vi "Quiz4.vi"() -> ()   [LabVIEW 2020]
uses:
  <vilib>/Platform/TimedLoop/XDataNode/timing_clust.ctl
  <vilib>/Platform/TimedLoop/XDataNode/nitl_modes.ctl
  <vilib>/Platform/TimedLoop/XDataNode/wakeup.ctl
  Control 1.ctl
  <vilib>/Utility/file.llb/Read Delimited Spreadsheet (string).vi
  <vilib>/platform/TimedLoop/XDataNode/XDataNode.xnode
  <vilib>/Platform/TimedLoop/XDataNode/XDNodeRunTimeDep.lvlib
panel:
  in  "OK Button 4":bool
  in  "OK Button 3":bool
  in  "Tab Control 2":enum32{"Login", "Registro", "Inicio"}(tab)
  in  "OK Button 2":bool
  in  "Clave 2":string
  in  "Usuario 2":string
  in  "Borrar usuario 2":string
  in  "Borrar 2":bool
  in  "Volver 2":bool
  in  "Agregar 2":bool
  in  "Clave Nueva 2":string
  in  "Nuevo Usuario 2":string
  out "concatenated string 2":string
  out "String 2":string="Usuario incorrecto"
  out "Usuarios Eliminados 2":string[](array[string])
  in  "Cerrar sesión 2":bool
  out "Usuarios 2":string[](array[string])
  out "Contraseñas 2":string[](array[string])
  out "Contraseñas":string[](array[string])
  out "Usuarios":string[](array[string])
  in  "Tab Control":enum32{"Login", "Registro", "Inicio"}(tab)
  in  "OK Button":bool
  in  "Clave":string
  in  "Usuario":string
  in  "Borrar usuario":string
  in  "Borrar":bool
  in  "Volver":bool
  in  "Agregar":bool
  in  "Clave Nueva":string
  in  "Nuevo Usuario":string
  out "concatenated string":string
  out "String":string="Usuario incorrecto"
  out "Usuarios Eliminados":string[](array[string])
  in  "Cerrar sesión":bool
  # "Usuario"
  # "Clave"
  # "Nuevo Usuario"
  # "Borrar usuario"
  # "Clave Nueva"
  # "Usuarios Eliminados"
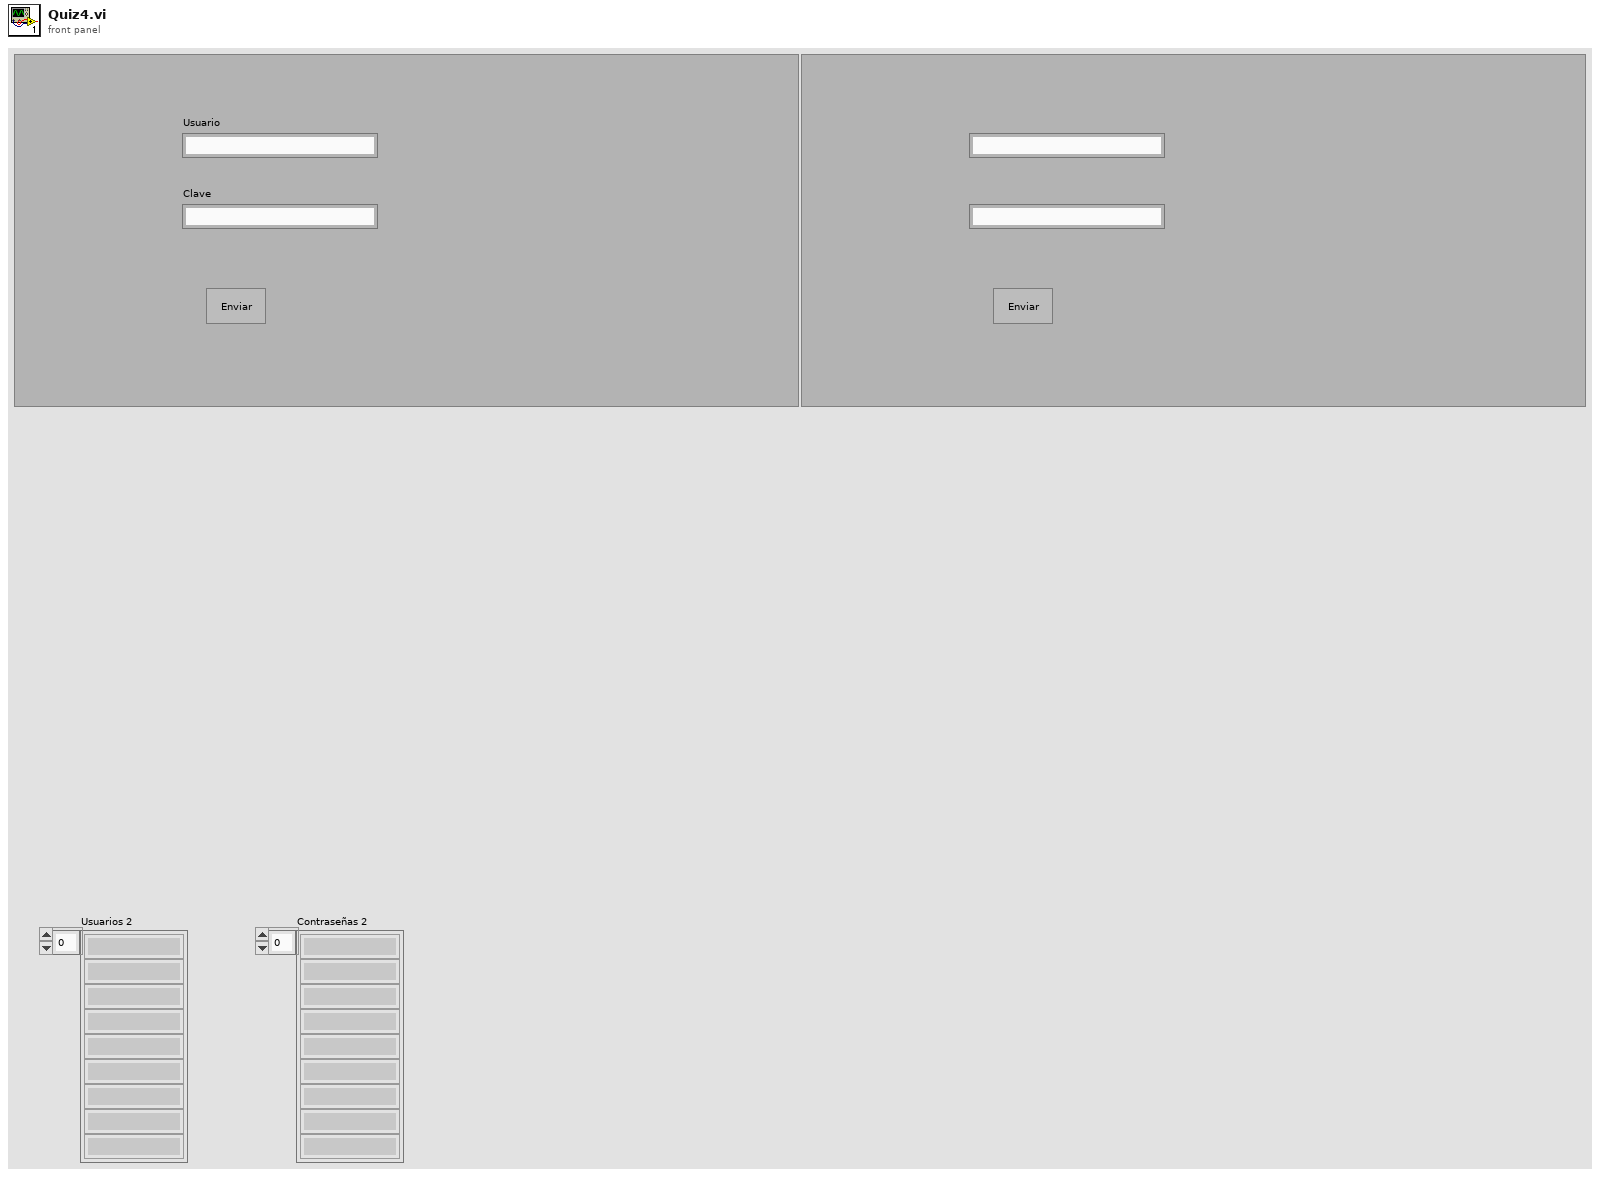
[diagram p1: front panel]
types:
  T1 = typedef "Control 1.ctl" = enum16{"Login", "Registro", "Inicio"}
  T2 = enum16{"open", "replace", "create", "open or create", "replace or create", "replace or create with confirmation"}
  T3 = typedef "XDNodeRunTimeDep.lvlib/timing_clust.ctl" = cluster{"Expected End [f-1]":u64, "Actual End [f-1]":u64, "Finished Late? [f-1]":bool, "Expected End [i-1]":u64, "Actual End [i-1]":u64, "Finished Late? [i-1]":bool, "Expected Start [i]":u64, "Actual Start [i]":u64, "Expected Start [f]":u64, "Actual Start [f]":u64, "Source Name":string, "Structure Name":string, "Period":i64, "Deadline":i64, "Offset":i64, "Start":i64, "Priority":i32, "Timeout":i32, "Mode":T4, "Wakeup Reason":T5, "Error":errorcluster, "Source Type":string, "Secondary Source Type":string, "Global End Time":u64, "Global Start Time":u64, "Frame Duration":u64, "Iteration Duration":u64, "Assigned CPU":i32, "I/O Scan Engine Mode":u32}
  T4 = typedef "XDNodeRunTimeDep.lvlib/nitl_modes.ctl" = enum32{"No Change", "Process missed periods, maintain original phase", "Discard missed periods, maintain original phase", "Process missed periods, ignore original phase", "Discard missed periods, ignore original phase"}
  T5 = typedef "XDNodeRunTimeDep.lvlib/wakeup.ctl" = enum32{"Normal", "Aborted", "Asynchronous wakeup", "Timing source error", "Timed loop error", "Timeout"}
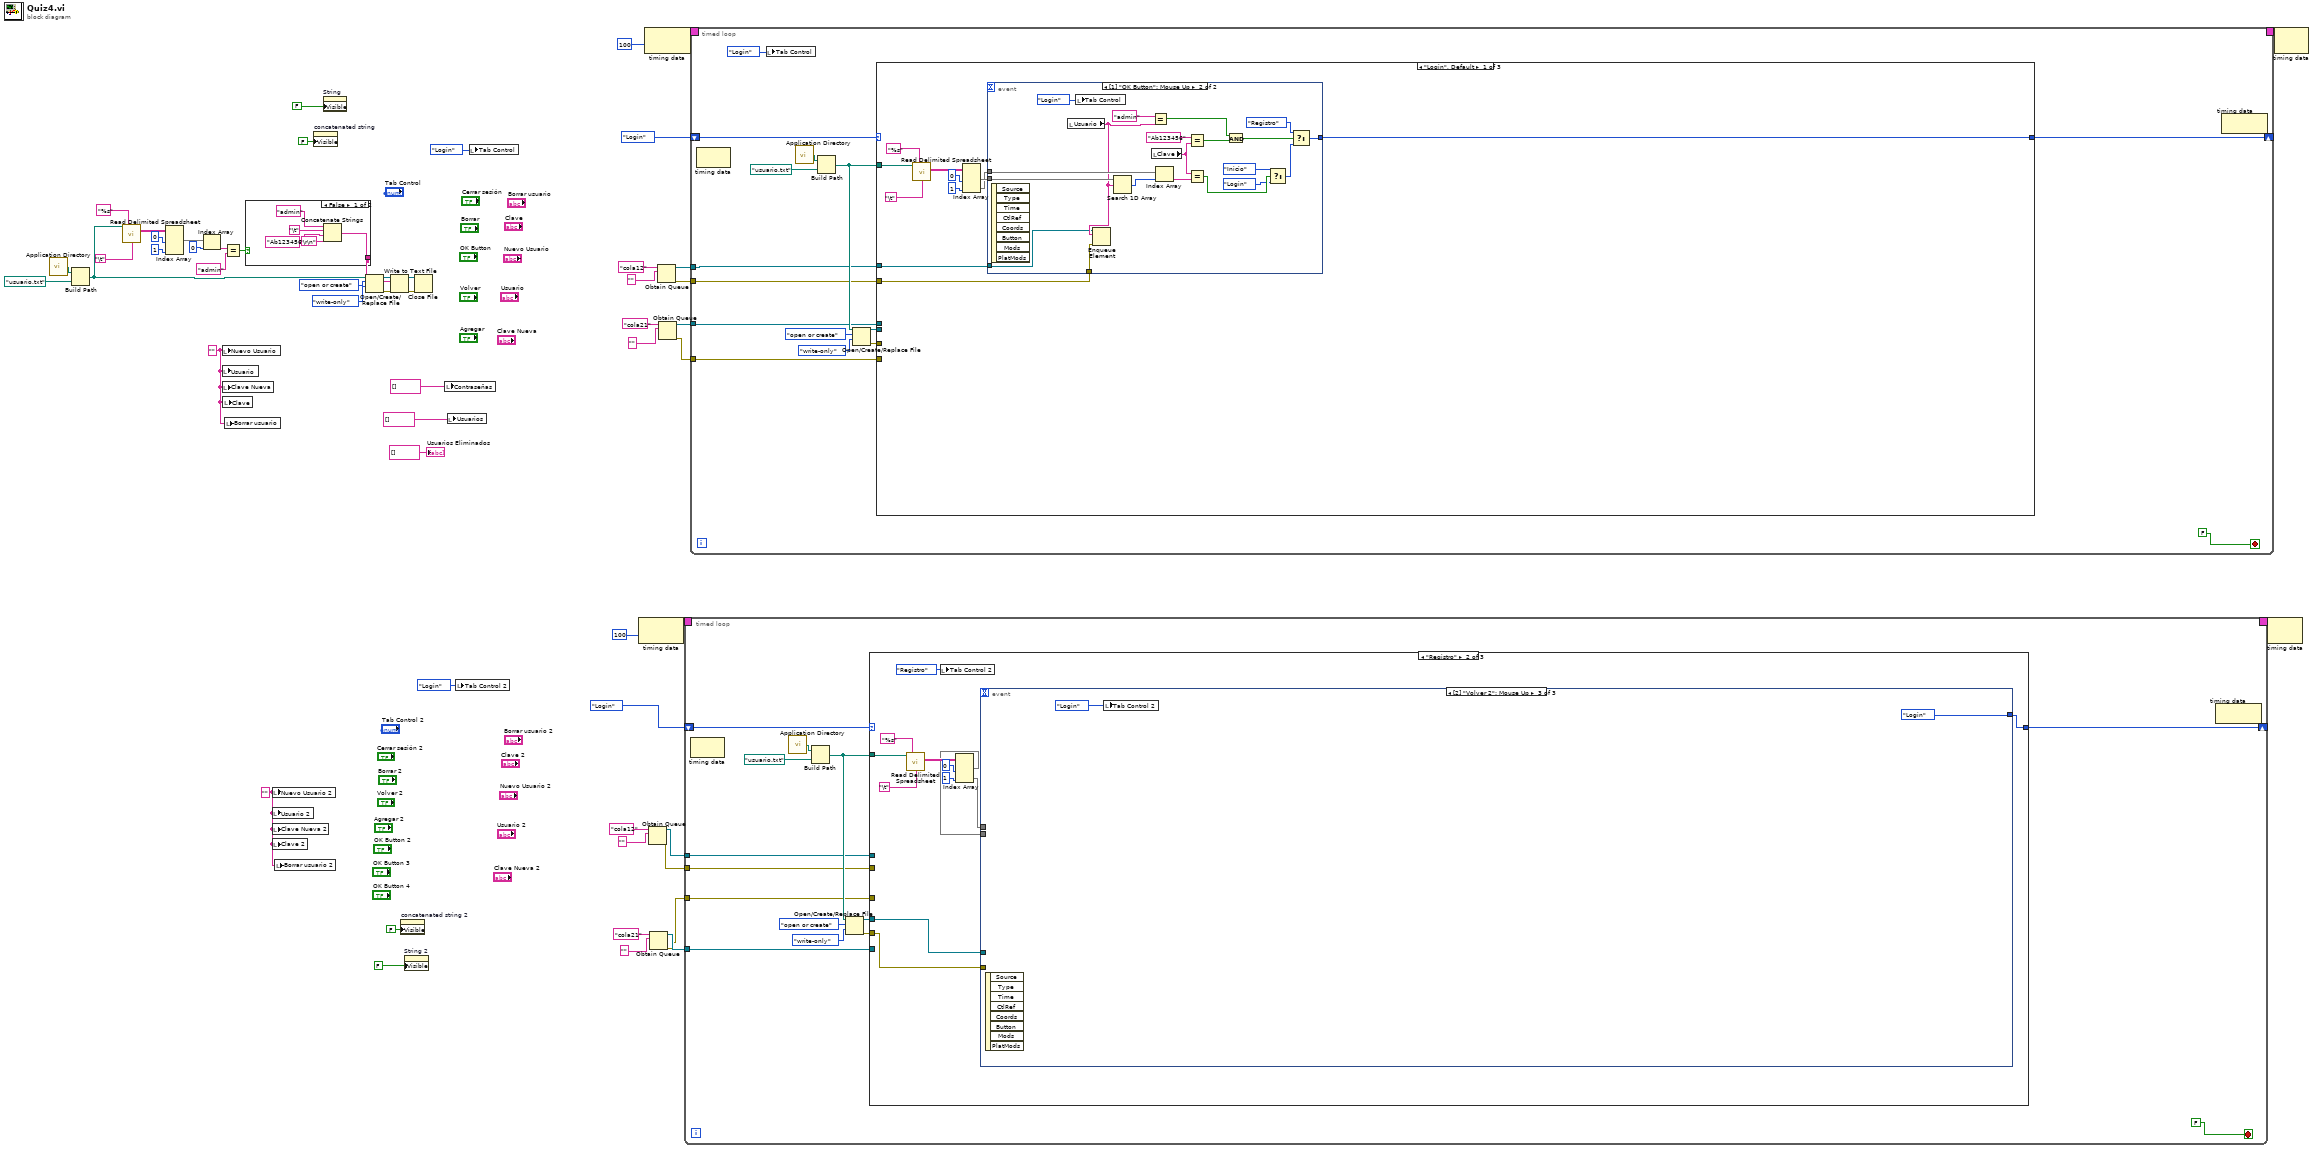
[diagram p0: block diagram]
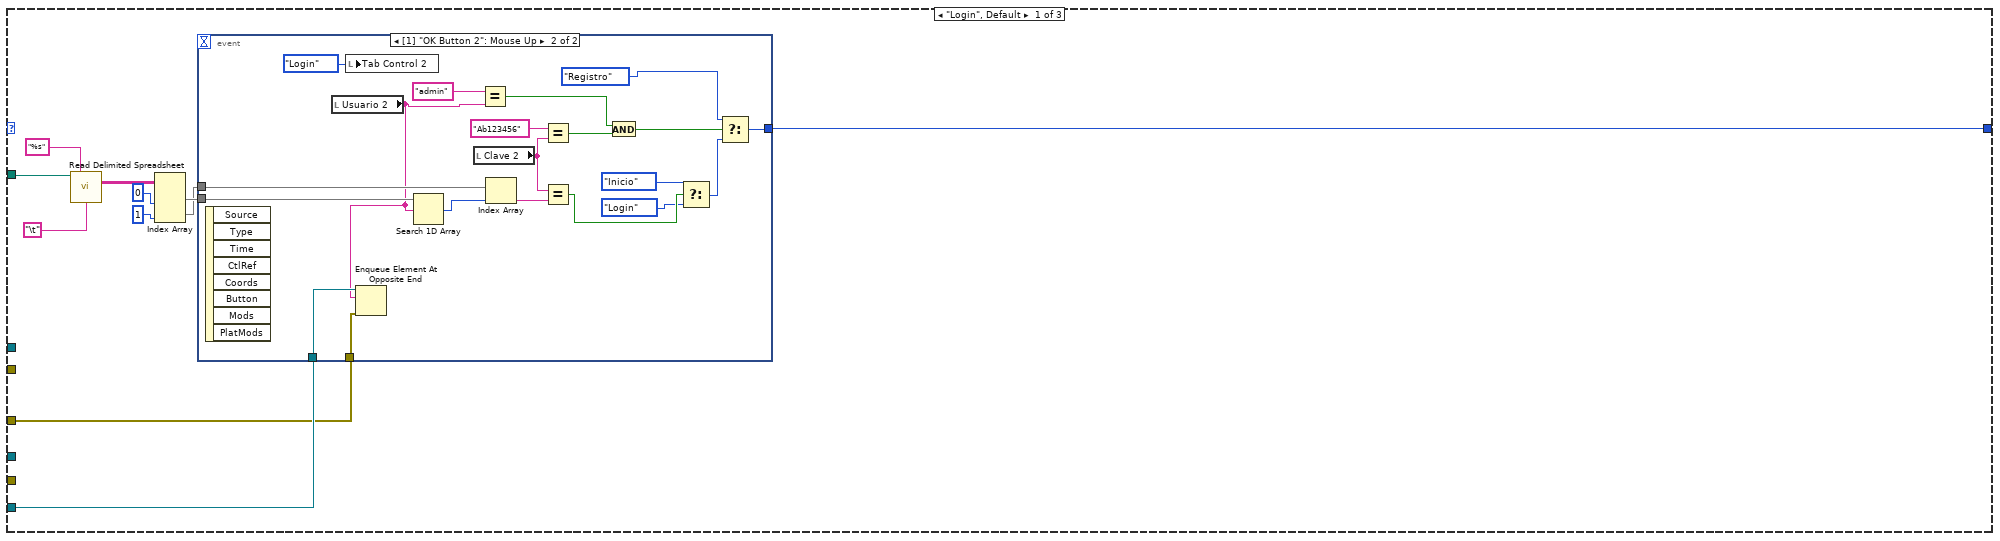
[diagram p2: hidden frame]
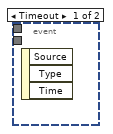
[diagram p3: hidden frame]
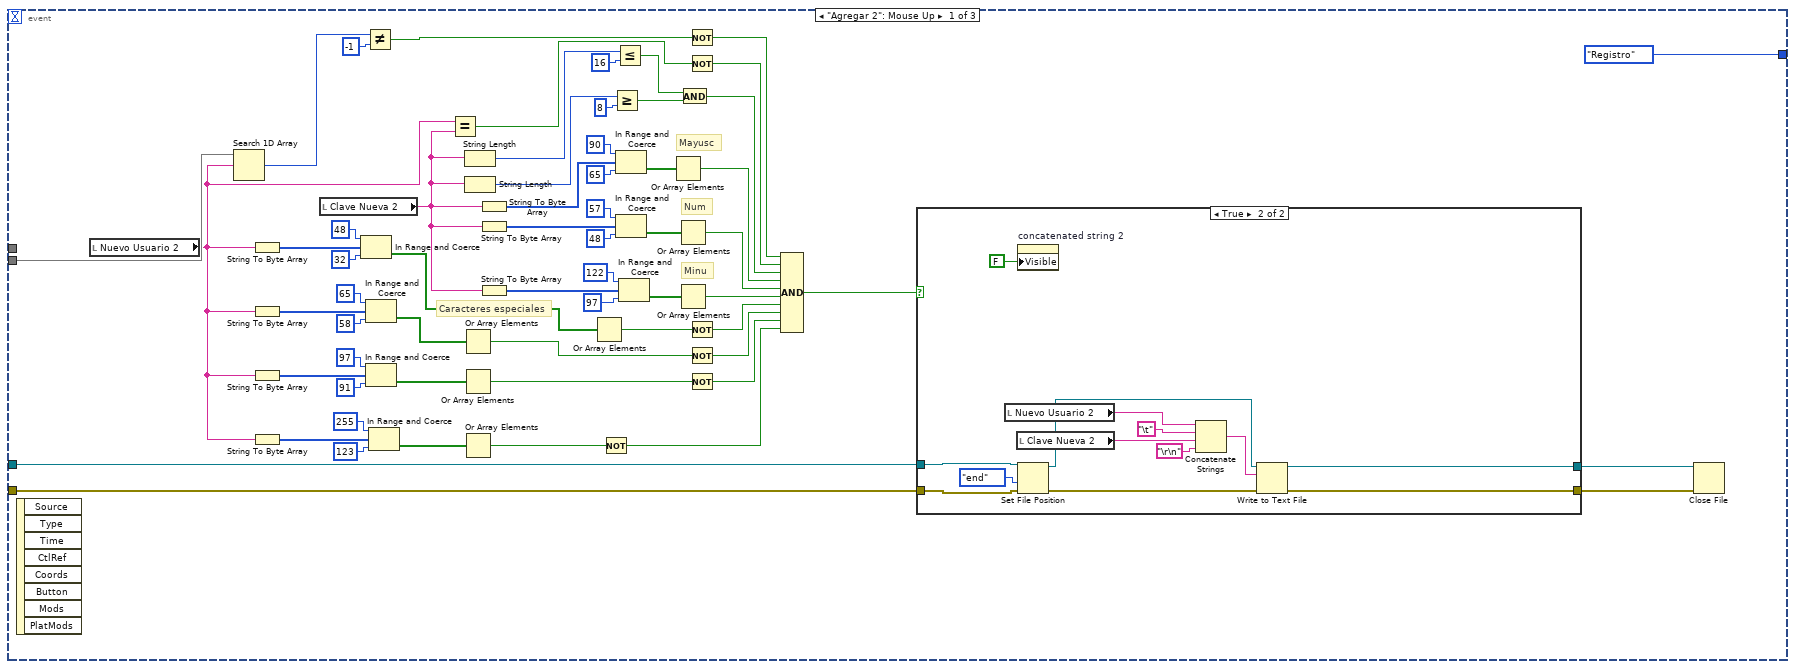
[diagram p4: hidden frame]
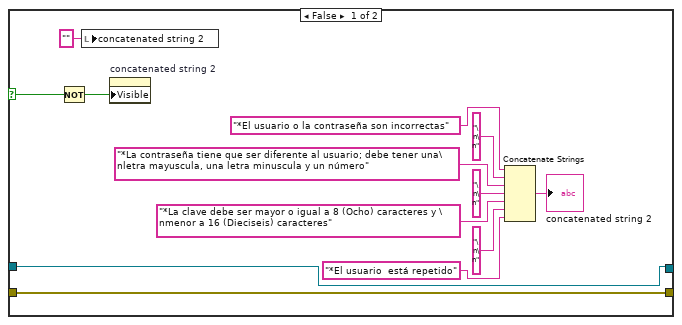
[diagram p5: hidden frame]
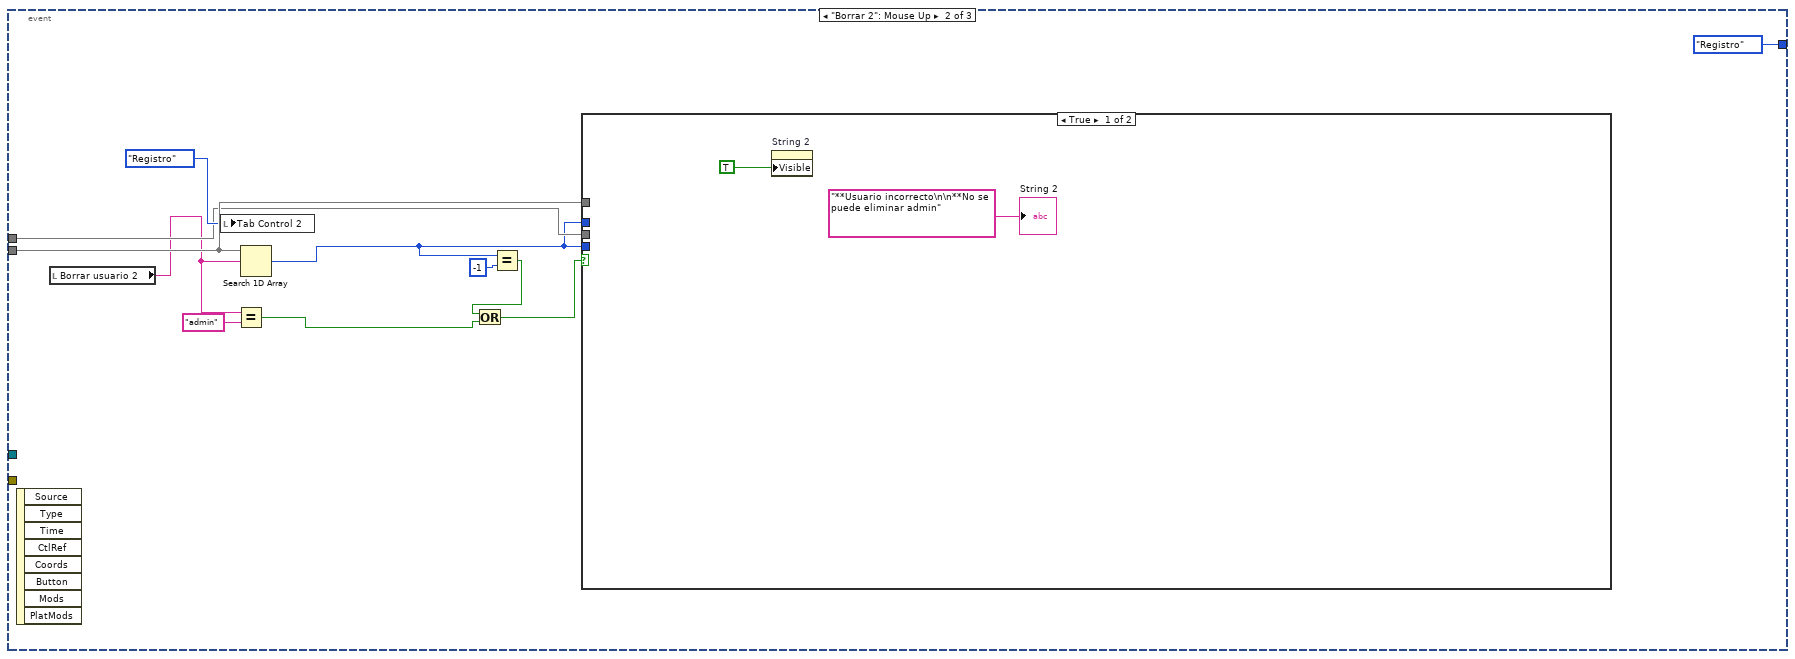
[diagram p6: hidden frame]
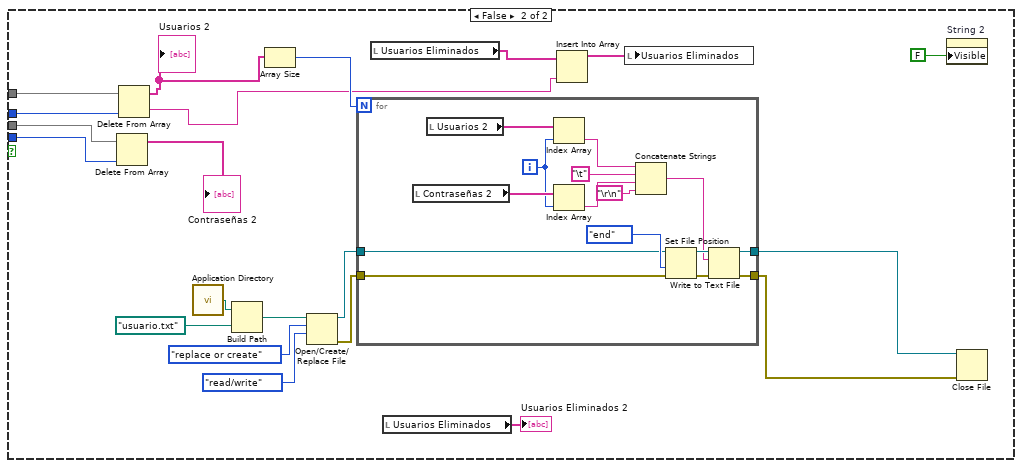
[diagram p7: hidden frame]
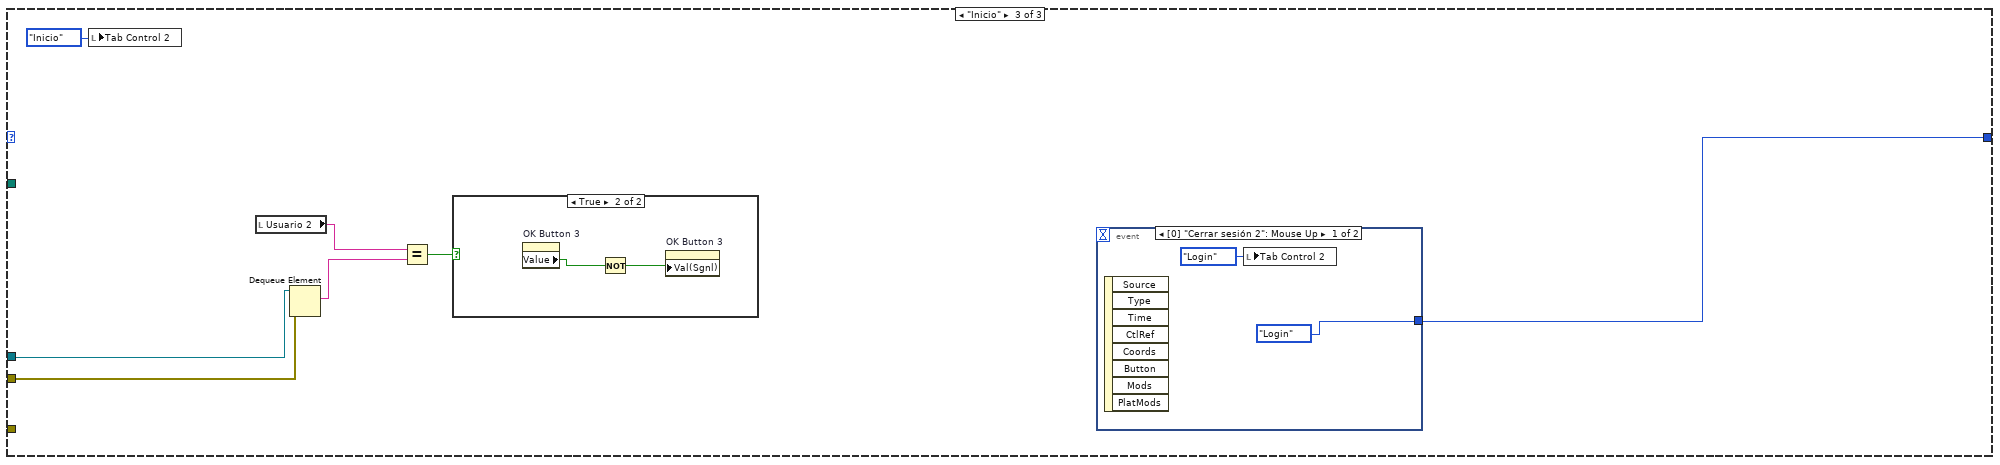
[diagram p8: hidden frame]
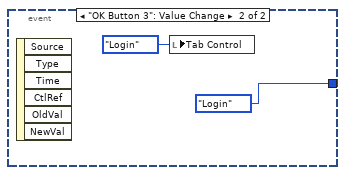
[diagram p10: hidden frame]
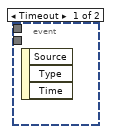
[diagram p12: hidden frame]
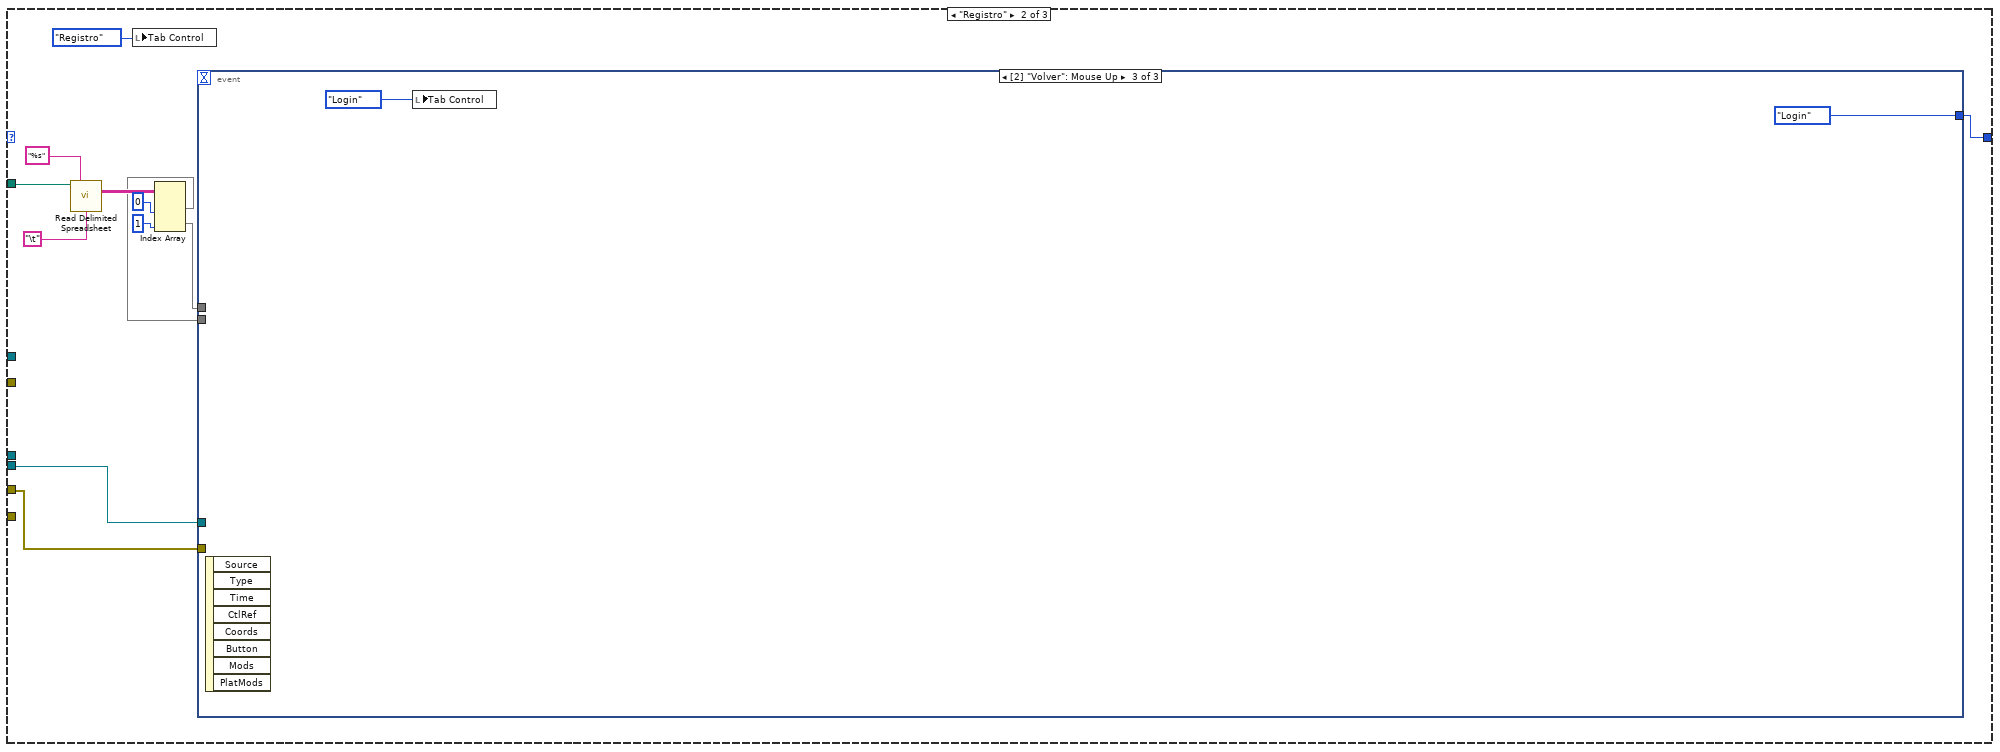
[diagram p13: hidden frame]
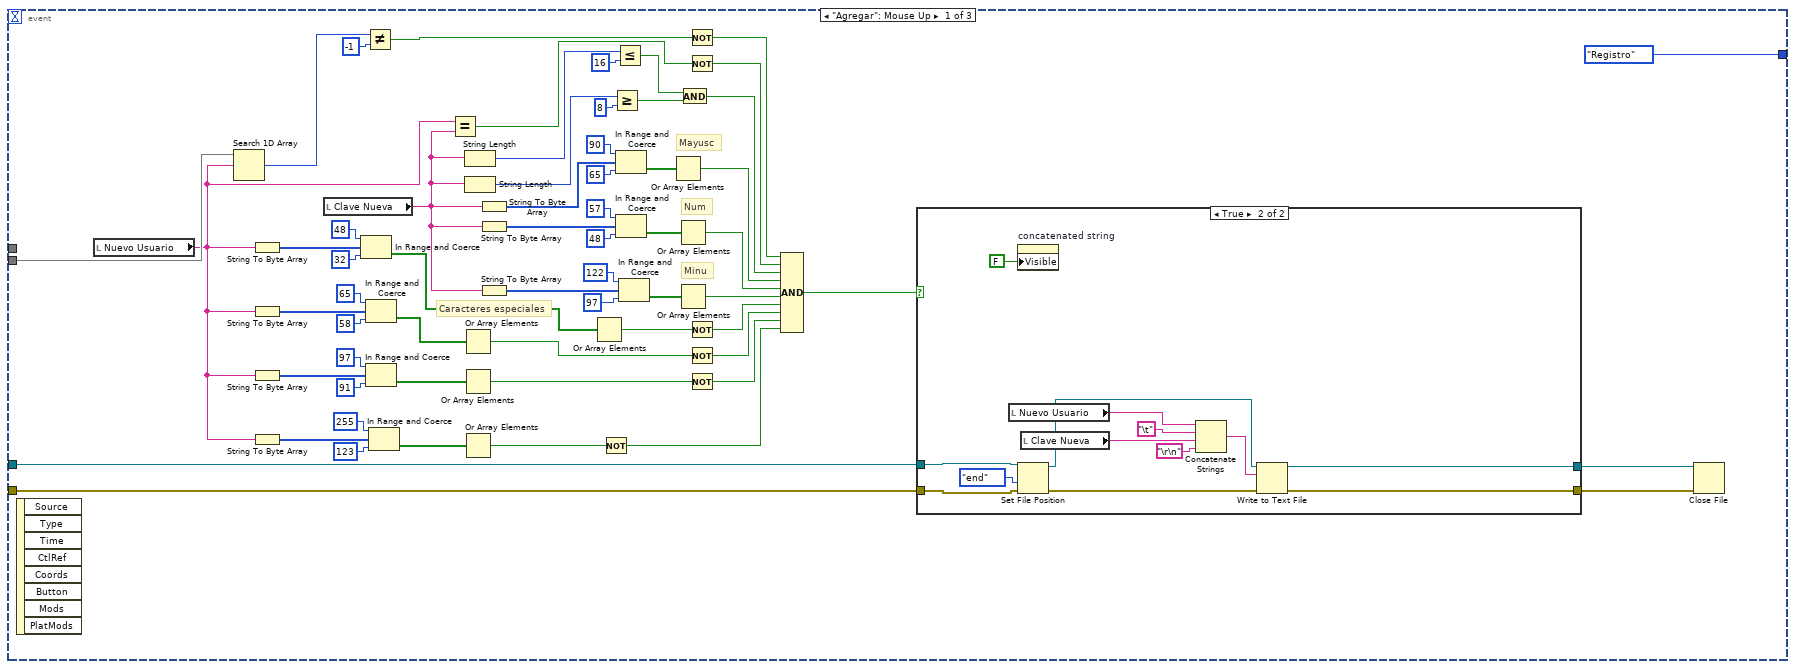
[diagram p14: hidden frame]
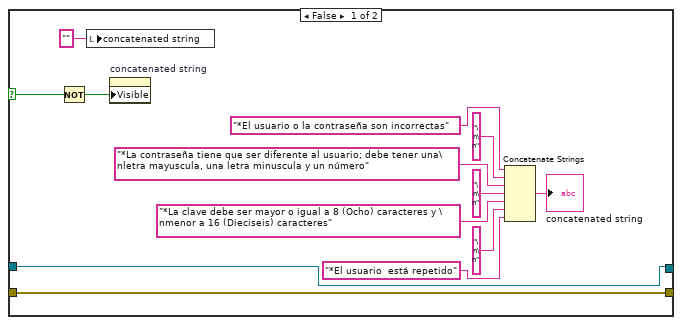
[diagram p15: hidden frame]
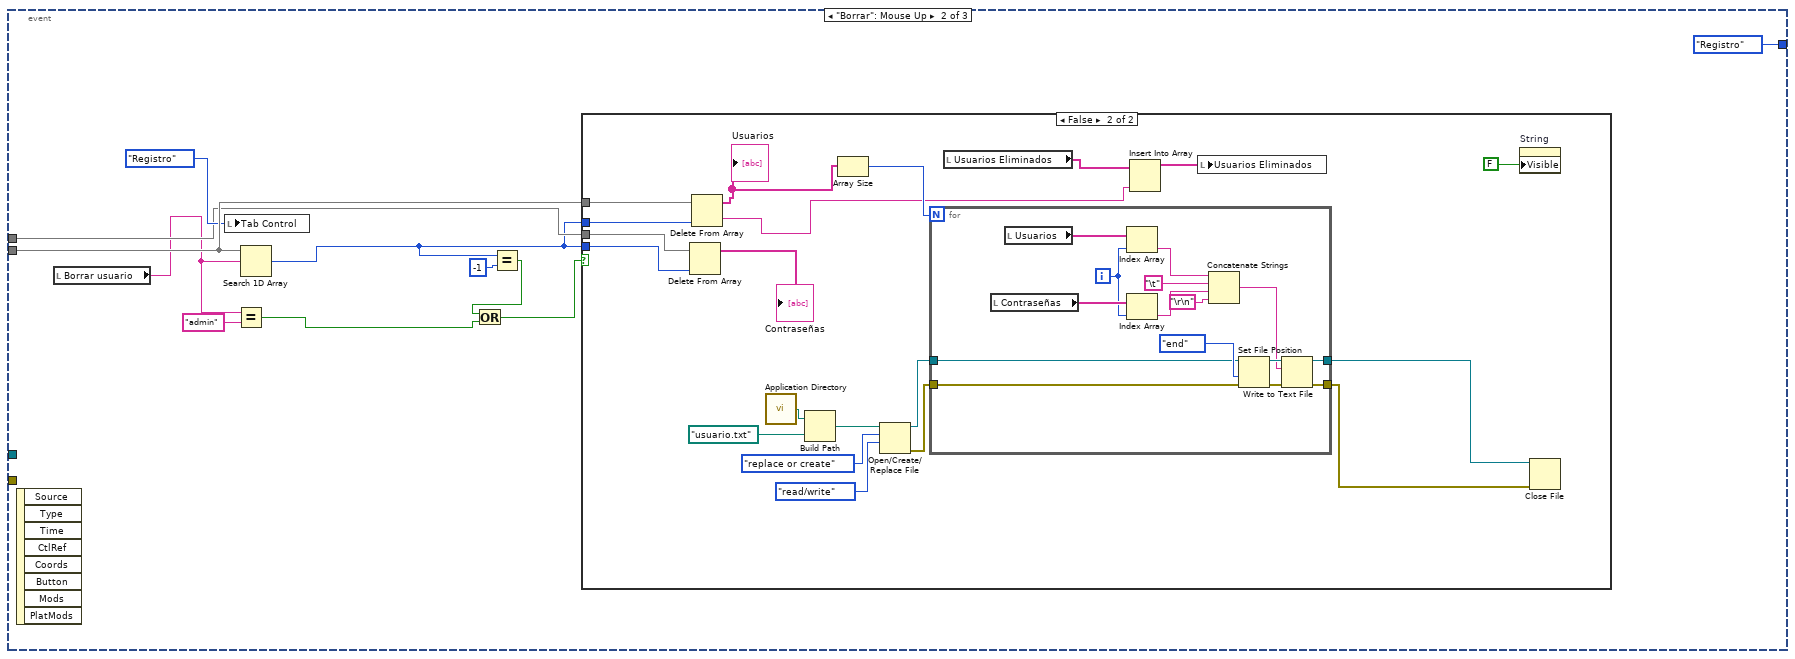
[diagram p16: hidden frame]
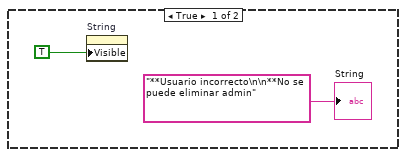
[diagram p17: hidden frame]
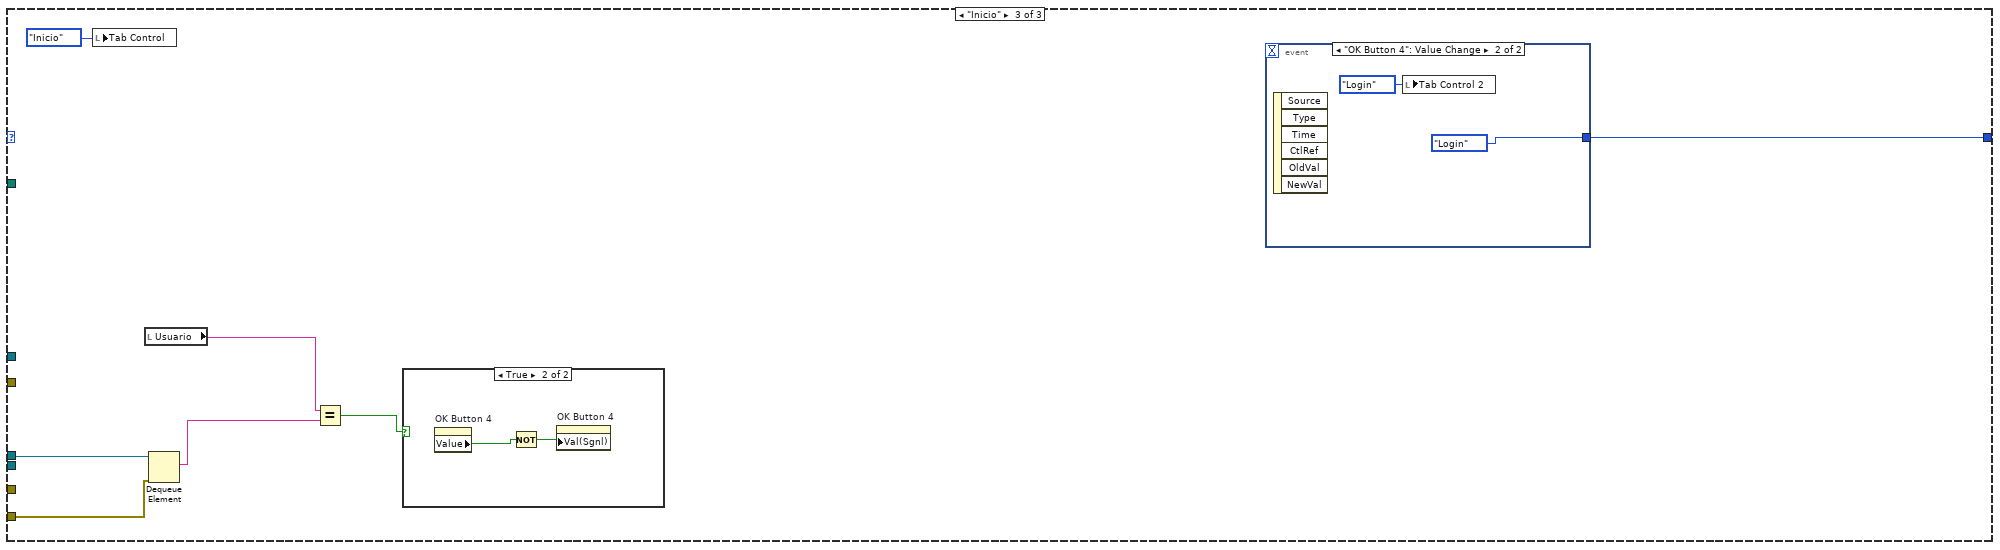
[diagram p18: hidden frame]
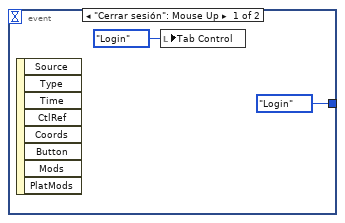
[diagram p20: hidden frame]
diagram:
  w20 = "" ("Nuevo Usuario")
  w25 = "" ("Nuevo Usuario")
  n1 = call <vilib>:"Application Directory.vi"() -> ("Application Directory"=w48:path)
  n2 = Build Path(base path=w48, name or relative path=path "usuario.txt" ("file path (use dialog)")) -> (appended path=w40:path)
  n3 = call-poly <vilib>:"Read Delimited Spreadsheet.vi"("file path (dialog if empty)"=w40, "format (%s)"="%s", "delimiter (\\t)"="\t") -> ("all rows"=w45:string[][])  [unwired: 7 in, 5 out]
  n4 = Index Array(array=w45, index (col) #1=0 ("disabled index (col)"), index (col) #2=1 ("index (col)")) -> (element #1=w39:string[])  [unwired: 2 in, 1 out]
  n5 = Index Array(array=w39, index=0) -> (element=w37:string)
  n6 = local write "Nuevo Usuario"(w25) -> ()
  n7 = local write "Usuario"(w25) -> ()
  n8 = local write "Clave Nueva"(w25) -> ()
  n9 = local write "Clave"(w25) -> ()
  n10 = Equal?(x=w37, y="admin") -> (x = y?=w35:bool)
  n11 = local write "Borrar usuario"(w25) -> ()
  n12 = case shown="False" w35 {
    tunnel: [w56 _] -> w30
    frame False {
      n13 = Concatenate Strings("admin" ("string"), "\t", "Ab123456" ("string"), "\r\n") -> (w56:string)
    }
    frame True {
    }
  }
  n14 = local write "Nuevo Usuario 2"(w20) -> ()
  n15 = local write "Usuario 2"(w20) -> ()
  n16 = local write "Clave Nueva 2"(w20) -> ()
  n17 = local write "Clave 2"(w20) -> ()
  n18 = local write "Borrar usuario 2"(w20) -> ()
  n19 = property on="concatenated string" class="Str"("Visible"=FALSE) -> ()  [unwired: 2 in, 2 out]
  n20 = property on="String" class="Str"("Visible"=FALSE) -> ()  [unwired: 2 in, 2 out]
  n21 = Open/Create/Replace File(file path (use dialog)=w40, operation (0:open)=T2."open or create", access (0:read/write)=enum16{"read/write", "read-only", "write-only"}."write-only") -> (refnum out=w34:refnum<file>, error out=w33:errorcluster)  [unwired: 3 in, 1 out]
  n22 = Write to Text File(file (use dialog)=w34, text=w30, error in=w33) -> (refnum out=w32:refnum<file>, error out=w31:errorcluster)  [unwired: 1 in, 1 out]
  n23 = property on="concatenated string 2" class="Str"("Visible"=FALSE) -> ()  [unwired: 2 in, 2 out]
  n24 = property on="String 2" class="Str"("Visible"=FALSE) -> ()  [unwired: 2 in, 2 out]
  n25 = Close File(refnum=w32, error in=w31) -> ()  [unwired: 2 out]
  n26 = local write "Contraseñas"(string[] [] ("array w/ subset deleted 2")) -> ()
  n27 = local write "Usuarios"(string[] [] ("array w/ subset deleted 2")) -> ()
  n28 = local write "Tab Control 2"(enum32{"Login", "Registro", "Inicio"}."Login" ("Tab Control 2")) -> ()
  n29 = local write "Tab Control"(enum32{"Login", "Registro", "Inicio"}."Login" ("Tab Control")) -> ()
  n30 = node-c288(i64 100 ("Period")) -> (w24:T3)
  n31 = node-c288(i64 100 ("Period")) -> (w55:T3)
  n32 = Obtain Queue(name (unnamed)="cola12", element data type="") -> (queue out=w11:refnum<queue>, error out=w10:errorcluster)  [unwired: 3 in, 1 out]
  n33 = Obtain Queue(name (unnamed)="cola21", element data type="") -> (queue out=w8:refnum<queue>, error out=w7:errorcluster)  [unwired: 3 in, 1 out]
  n34 = Obtain Queue(name (unnamed)="cola12", element data type="") -> (queue out=w15:refnum<queue>, error out=w14:errorcluster)  [unwired: 3 in, 1 out]
  n35 = Obtain Queue(name (unnamed)="cola21", element data type="") -> (queue out=w5:refnum<queue>, error out=w4:errorcluster)  [unwired: 3 in, 1 out]
  n36 = timed-loop {
    timing: w24 -> [_]
    timing-out: [_] -> w23
    shift-right: [w73] -> _
    shift-left: Control_1."Login" -> [w61]
    tunnel: w11 -> [w65]
    tunnel: w10 -> [w64]
    tunnel: w8 -> [w63]
    tunnel: w7 -> [w62]
    stop <- FALSE stop-if-true
    n37 = node-c288() -> ()  [unwired: 1 in, 1 out]
    n38 = call <vilib>:"Application Directory.vi"() -> ("Application Directory"=w71:path)
    n39 = Build Path(base path=w71, name or relative path=path "usuario.txt" ("file path (use dialog)")) -> (appended path=w66:path)
    n40 = Open/Create/Replace File(file path (use dialog)=w66, operation (0:open)=T2."open or create", access (0:read/write)=enum16{"read/write", "read-only", "write-only"}."write-only") -> (refnum out=w69:refnum<file>, error out=w68:errorcluster)  [unwired: 3 in, 1 out]
    n41 = case shown="\"Registro\"" w61 {
      tunnel: [w85 w114 w261] -> w73
      tunnel: w69 -> [_ w116 _]
      tunnel: w68 -> [_ w115 _]
      tunnel: w66 -> [w79 w111 _]
      tunnel: w65 -> [_ _ w260]
      tunnel: w64 -> [_ _ w259]
      tunnel: w63 -> [w76 _ _]
      tunnel: w62 -> [w75 _ _]
      frame "Login", Default {
        n42 = call-poly <vilib>:"Read Delimited Spreadsheet.vi"("file path (dialog if empty)"=w79, "format (%s)"="%s", "delimiter (\\t)"="\t") -> ("all rows"=w80:string[][])  [unwired: 7 in, 5 out]
        n43 = Index Array(array=w80, index (col) #1=0 ("disabled index (col)"), index (col) #2=1 ("index (col)")) -> (element #1=w78:string[], element #2=w77:string[])  [unwired: 2 in]
        n44 = event shown="[1] \"OK Button 2\": Mouse Up" {
          selector: _ -> [_ _]
          dyn-events: _ -> [_ _]
          timeout: _ -> [_ _]
          tunnel: [_ w100] -> w85
          tunnel: w78 -> [_ w98]
          tunnel: w77 -> [_ w97]
          tunnel: w76 -> [_ w89]
          tunnel: w75 -> [_ w88]
          event Timeout {
            n45 = event-data() -> ()  [unwired: 1 in, 3 out]
          }
          event "OK Button 2": Mouse Up {
            n46 = event-data() -> ()  [unwired: 1 in, 8 out]
            n47 = local read "Usuario 2"() -> (w87:string)
            n48 = local write "Tab Control 2"(enum32{"Login", "Registro", "Inicio"}."Login" ("Tab Control")) -> ()
            n49 = Enqueue Element At Opposite End(queue=w89, element=w87, error in (no error)=w88) -> ()  [unwired: 1 in, 3 out]
            n50 = Search 1D Array(1D array=w98, element=w87) -> (index of element=w96:i32)  [unwired: 1 in]
            n51 = local read "Clave 2"() -> (w95:string)
            n52 = Equal?(x="admin", y=w87) -> (x = y?=w103:bool)
            n53 = Index Array(array=w97, index=w96) -> (element=w94:string)
            n54 = Equal?(x="Ab123456", y=w95) -> (x = y?=w102:bool)
            n55 = Equal?(x=w95, y=w94) -> (x = y?=w93:bool)
            n56 = And(x=w103, y=w102) -> (x .and. y?=w101:bool)
            n57 = Select(t=Control_1."Inicio", s=w93, f=Control_1."Login") -> (s? t:f=w90:T1)
            n58 = Select(t=Control_1."Registro", s=w101, f=w90) -> (s? t:f=w100:T1)
          }
        }
      }
      frame "Registro" {
        n59 = call-poly <vilib>:"Read Delimited Spreadsheet.vi"("file path (dialog if empty)"=w111, "format (%s)"="%s", "delimiter (\\t)"="\t") -> ("all rows"=w108:string[][])  [unwired: 7 in, 5 out]
        n60 = local write "Tab Control 2"(enum32{"Login", "Registro", "Inicio"}."Registro" ("Tab Control")) -> ()
        n61 = Index Array(array=w108, index (col) #1=0 ("disabled index (col)"), index (col) #2=1 ("index (col)")) -> (element #1=w107:string[], element #2=w106:string[])  [unwired: 2 in]
        n62 = event shown="[2] \"Volver 2\": Mouse Up" {
          selector: _ -> [_ _ _]
          dyn-events: _ -> [_ _ _]
          timeout: _ -> [_ _ _]
          tunnel: w116 -> [w151 _ _]
          tunnel: w115 -> [w150 _ _]
          tunnel: [Control_1."Registro" Control_1."Registro" Control_1."Login"] -> w114
          tunnel: w107 -> [w147 w215 _]
          tunnel: w106 -> [_ w212 _]
          event "Agregar 2": Mouse Up {
            # "Caracteres especiales"
            # "Minu"
            # "Num"
            # "Mayusc"
            n63 = event-data() -> ()  [unwired: 1 in, 8 out]
            n64 = local read "Nuevo Usuario 2"() -> (w126:string)
            n65 = Search 1D Array(1D array=w147, element=w126) -> (index of element=w146:i32)  [unwired: 1 in]
            n66 = String To Byte Array(string=w126) -> (unsigned byte array=w142:u8[])
            n67 = String To Byte Array(string=w126) -> (unsigned byte array=w137:u8[])
            n68 = String To Byte Array(string=w126) -> (unsigned byte array=w136:u8[])
            n69 = String To Byte Array(string=w126) -> (unsigned byte array=w127:u8[])
            n70 = local read "Clave Nueva 2"() -> (w148:string)
            n71 = In Range and Coerce(upper limit=u8 48, x=w142, lower limit=u8 32) -> (In Range?=w133:bool[])  [unwired: 1 out]
            n72 = Not Equal?(x=w146, y=-1) -> (x != y?=w144:bool)
            n73 = In Range and Coerce(upper limit=u8 65, x=w137, lower limit=u8 58) -> (In Range?=w132:bool[])  [unwired: 1 out]
            n74 = In Range and Coerce(upper limit=u8 97, x=w136, lower limit=u8 91) -> (In Range?=w131:bool[])  [unwired: 1 out]
            n75 = In Range and Coerce(upper limit=u8 255, x=w127, lower limit=u8 123) -> (In Range?=w130:bool[])  [unwired: 1 out]
            n76 = Equal?(x=w126, y=w148) -> (x = y?=w156:bool)
            n77 = Or Array Elements(Boolean array=w132) -> (logical OR=w124:bool)
            n78 = Or Array Elements(Boolean array=w131) -> (logical OR=w123:bool)
            n79 = Or Array Elements(Boolean array=w130) -> (logical OR=w122:bool)
            n80 = String Length(string=w148) -> (length=w178:i32)
            n81 = String Length(string=w148) -> (length=w176:i32)
            n82 = String To Byte Array(string=w148) -> (unsigned byte array=w164:u8[])
            n83 = String To Byte Array(string=w148) -> (unsigned byte array=w165:u8[])
            n84 = String To Byte Array(string=w148) -> (unsigned byte array=w172:u8[])
            n85 = Or Array Elements(Boolean array=w133) -> (logical OR=w125:bool)
            n86 = Not(x=w122) -> (.not. x?=w118:bool)
            n87 = Greater Or Equal?(x=w176, y=8) -> (x >= y?=w173:bool)
            n88 = Less Or Equal?(x=w178, y=16) -> (x <= y?=w174:bool)
            n89 = In Range and Coerce(upper limit=u8 90, x=w164, lower limit=u8 65) -> (In Range?=w161:bool[])  [unwired: 1 out]
            n90 = In Range and Coerce(upper limit=u8 57, x=w165, lower limit=u8 48) -> (In Range?=w168:bool[])  [unwired: 1 out]
            n91 = In Range and Coerce(upper limit=u8 122, x=w172, lower limit=u8 97) -> (In Range?=w169:bool[])  [unwired: 1 out]
            n92 = Or Array Elements(Boolean array=w161) -> (logical OR=w159:bool)
            n93 = Or Array Elements(Boolean array=w168) -> (logical OR=w158:bool)
            n94 = Or Array Elements(Boolean array=w169) -> (logical OR=w157:bool)
            n95 = And(x=w174, y=w173) -> (x .and. y?=w160:bool)
            n96 = Not(x=w144) -> (.not. x?=w143:bool)
            n97 = Not(x=w156) -> (.not. x?=w155:bool)
            n98 = Not(x=w125) -> (.not. x?=w121:bool)
            n99 = Not(x=w124) -> (.not. x?=w120:bool)
            n100 = Not(x=w123) -> (.not. x?=w119:bool)
            n101 = Compound Arithmetic op=AND(w143, w155, w160, w159, w158, w157, w121, w120, w119, w118) -> (w154:bool)
            n102 = case shown="True" w154 {
              selector: w154 -> [w187 _]
              tunnel: [w182 w196] -> w153
              tunnel: [w181 w195] -> w152
              tunnel: w151 -> [w182 w193]
              tunnel: w150 -> [w181 w192]
              frame False {
                n103 = Not(x=w187) -> (.not. x?=w186:bool)
                n104 = local write "concatenated string 2"("" ("concatenated string")) -> ()
                n105 = property on="concatenated string 2" class="Str"("Visible"=w186) -> ()  [unwired: 2 in, 2 out]
                n106 = Concatenate Strings("*El usuario o la contraseña son incorrectas", "\n\n" ("string"), "*La contraseña tiene que ser diferente al usuario; debe tener una\nletra mayuscula, una letra minuscula y un número", "\n\n" ("string"), "*La clave debe ser mayor o igual a 8 (Ocho) caracteres y \nmenor a 16 (Dieciseis) caracteres", "\n\n" ("string"), "*El usuario  está repetido") -> (→"concatenated string 2":string)
              }
              frame True {
                n107 = local read "Nuevo Usuario 2"() -> (w199:string)
                n108 = local read "Clave Nueva 2"() -> (w200:string)
                n109 = property on="concatenated string 2" class="Str"("Visible"=FALSE) -> ()  [unwired: 2 in, 2 out]
                n110 = Set File Position(refnum=w193, from (0:start)=enum16{"start", "end", "current"}."end", error in=w192) -> (refnum out=w197:refnum<file>, error out=w202:errorcluster)  [unwired: 1 in]
                n111 = Concatenate Strings(w199, "\t", w200, "\r\n") -> (w203:string)
                n112 = Write to Text File(file (use dialog)=w197, text=w203, error in=w202) -> (refnum out=w196:refnum<file>, error out=w195:errorcluster)  [unwired: 1 in, 1 out]
              }
            }
            n113 = Close File(refnum=w153, error in=w152) -> ()  [unwired: 2 out]
          }
          event "Borrar 2": Mouse Up {
            n114 = event-data() -> ()  [unwired: 1 in, 8 out]
            n115 = local read "Borrar usuario 2"() -> (w205:string)
            n116 = local write "Tab Control 2"(enum32{"Login", "Registro", "Inicio"}."Registro" ("Tab Control")) -> ()
            n117 = Equal?(x=w205, y="admin") -> (x = y?=w206:bool)
            n118 = Search 1D Array(1D array=w215, element=w205) -> (index of element=w210:i32)  [unwired: 1 in]
            n119 = Equal?(x=w210, y=-1) -> (x = y?=w208:bool)
            n120 = Or(x=w208, y=w206) -> (x .or. y?=w207:bool)
            n121 = case shown="True" w207 {
              tunnel: w215 -> [_ w238]
              tunnel: w212 -> [_ w237]
              tunnel: w210 -> [_ w236]
              tunnel: w210 -> [_ w235]
              frame True {
                n122 = property on="String 2" class="Str"("Visible"=TRUE) -> ()  [unwired: 2 in, 2 out]
                "String 2" <- "**Usuario incorrecto\n\n**No se puede eliminar admin"
              }
              frame False {
                n123 = Delete From Array(array=w237, index=w236) -> (array with subset deleted=→"Contraseñas 2":string[])  [unwired: 1 in, 1 out]
                n124 = Delete From Array(array=w238, index=w235) -> (deleted portion=w220:string, array with subset deleted=w232:string[])  [unwired: 1 in]
                "Usuarios 2" <- w232
                n125 = call <vilib>:"Application Directory.vi"() -> ("Application Directory"=w225:path)
                n126 = Build Path(base path=w225, name or relative path=path "usuario.txt" ("file path (use dialog)")) -> (appended path=w226:path)
                n127 = Array Size(array=w232) -> (size(s)=w231:i32)
                n128 = Open/Create/Replace File(file path (use dialog)=w226, operation (0:open)=T2."replace or create", access (0:read/write)=enum16{"read/write", "read-only", "write-only"}."read/write") -> (refnum out=w223:refnum<file>, error out=w222:errorcluster)  [unwired: 3 in, 1 out]
                n129 = for {
                  N: w231 -> [_]
                  tunnel: [w242] -> w229
                  tunnel: [w241] -> w230
                  tunnel: w223 -> [w240]
                  tunnel: w222 -> [w239]
                  i -> [w251]
                  n130 = local read "Contraseñas 2"() -> (w252:string[])
                  n131 = local read "Usuarios 2"() -> (w253:string[])
                  n132 = Index Array(array=w253, index=w251) -> (element=w244:string)
                  n133 = Index Array(array=w252, index=w251) -> (element=w243:string)
                  n134 = Concatenate Strings(w244, "\t", w243, "\r\n") -> (w246:string)
                  n135 = Set File Position(refnum=w240, from (0:start)=enum16{"start", "end", "current"}."end", error in=w239) -> (refnum out=w248:refnum<file>, error out=w250:errorcluster)  [unwired: 1 in]
                  n136 = Write to Text File(file (use dialog)=w248, text=w246, error in=w250) -> (refnum out=w241:refnum<file>, error out=w242:errorcluster)  [unwired: 1 in, 1 out]
                }
                n137 = local read "Usuarios Eliminados"() -> (w221:string[])
                n138 = local read "Usuarios Eliminados"() -> (→"Usuarios Eliminados 2":string[])
                n139 = Insert Into Array(array=w221, new element=w220) -> (w219:string[])  [unwired: 1 in]
                n140 = local write "Usuarios Eliminados"(w219) -> ()
                n141 = property on="String 2" class="Str"("Visible"=FALSE) -> ()  [unwired: 2 in, 2 out]
                n142 = Close File(refnum=w230, error in=w229) -> ()  [unwired: 2 out]
              }
            }
          }
          event "Volver 2": Mouse Up {
            n143 = event-data() -> ()  [unwired: 1 in, 8 out]
            n144 = local write "Tab Control 2"(enum32{"Login", "Registro", "Inicio"}."Login" ("Tab Control")) -> ()
          }
        }
      }
      frame "Inicio" {
        n145 = local write "Tab Control 2"(enum32{"Login", "Registro", "Inicio"}."Inicio" ("Tab Control")) -> ()
        n146 = local read "Usuario 2"() -> (w258:string)
        n147 = Dequeue Element(queue=w260, error in (no error)=w259) -> (element=w257:string)  [unwired: 1 in, 3 out]
        n148 = Equal?(x=w258, y=w257) -> (x = y?=w256:bool)
        n149 = case shown="True" w256 {
          frame False {
          }
          frame True {
            n150 = property on="OK Button 3" class="Bool (strict)"() -> ("Value"=w264:bool)  [unwired: 2 in, 2 out]
            n151 = Not(x=w264) -> (.not. x?=w263:bool)
            n152 = property on="OK Button 3" class="Bool (strict)"("Val(Sgnl)"=w263) -> ()  [unwired: 2 in, 2 out]
          }
        }
        n153 = event shown="[0] \"Cerrar sesión 2\": Mouse Up" {
          selector: _ -> [_ _]
          dyn-events: _ -> [_ _]
          timeout: _ -> [_ _]
          tunnel: [Control_1."Login" Control_1."Login"] -> w261
          event "Cerrar sesión 2": Mouse Up {
            n154 = event-data() -> ()  [unwired: 1 in, 8 out]
            n155 = local write "Tab Control 2"(enum32{"Login", "Registro", "Inicio"}."Login" ("Tab Control")) -> ()
          }
          event "OK Button 3": Value Change {
            n156 = event-data() -> ()  [unwired: 1 in, 6 out]
            n157 = local write "Tab Control"(enum32{"Login", "Registro", "Inicio"}."Login" ("Tab Control")) -> ()
          }
        }
      }
    }
    n158 = node-c288() -> ()  [unwired: 1 in, 1 out]
  }
  n159 = timed-loop {
    timing: w55 -> [_]
    timing-out: [_] -> w54
    shift-right: [w283] -> _
    shift-left: Control_1."Login" -> [w284]
    tunnel: w15 -> [w275]
    tunnel: w14 -> [w274]
    tunnel: w5 -> [w273]
    tunnel: w4 -> [w272]
    stop <- FALSE stop-if-true
    n160 = node-c288() -> ()  [unwired: 1 in, 1 out]
    n161 = local write "Tab Control"(enum32{"Login", "Registro", "Inicio"}."Login" ("Tab Control")) -> ()
    n162 = call <vilib>:"Application Directory.vi"() -> ("Application Directory"=w281:path)
    n163 = Build Path(base path=w281, name or relative path=path "usuario.txt" ("file path (use dialog)")) -> (appended path=w276:path)
    n164 = Open/Create/Replace File(file path (use dialog)=w276, operation (0:open)=T2."open or create", access (0:read/write)=enum16{"read/write", "read-only", "write-only"}."write-only") -> (refnum out=w279:refnum<file>, error out=w278:errorcluster)  [unwired: 3 in, 1 out]
    n165 = case shown="\"Login\", Default" w284 {
      tunnel: [w296 w325 w471] -> w283
      tunnel: w279 -> [_ w327 _]
      tunnel: w278 -> [_ w326 _]
      tunnel: w276 -> [w290 w322 _]
      tunnel: w275 -> [w287 _ _]
      tunnel: w274 -> [w286 _ _]
      tunnel: w273 -> [_ _ w470]
      tunnel: w272 -> [_ _ w469]
      frame "Login", Default {
        n166 = call-poly <vilib>:"Read Delimited Spreadsheet.vi"("file path (dialog if empty)"=w290, "format (%s)"="%s", "delimiter (\\t)"="\t") -> ("all rows"=w291:string[][])  [unwired: 7 in, 5 out]
        n167 = Index Array(array=w291, index (col) #1=0 ("disabled index (col)"), index (col) #2=1 ("index (col)")) -> (element #1=w289:string[], element #2=w288:string[])  [unwired: 2 in]
        n168 = event shown="[1] \"OK Button\": Mouse Up" {
          selector: _ -> [_ _]
          dyn-events: _ -> [_ _]
          timeout: _ -> [_ _]
          tunnel: [_ w310] -> w296
          tunnel: w289 -> [_ w308]
          tunnel: w288 -> [_ w307]
          tunnel: w287 -> [_ w298]
          tunnel: w286 -> [_ w297]
          event Timeout {
            n169 = event-data() -> ()  [unwired: 1 in, 3 out]
          }
          event "OK Button": Mouse Up {
            n170 = event-data() -> ()  [unwired: 1 in, 8 out]
            n171 = local read "Usuario"() -> (w299:string)
            n172 = local write "Tab Control"(enum32{"Login", "Registro", "Inicio"}."Login" ("Tab Control")) -> ()
            n173 = Enqueue Element(queue=w298, element=w299, error in (no error)=w297) -> ()  [unwired: 1 in, 3 out]
            n174 = Search 1D Array(1D array=w308, element=w299) -> (index of element=w306:i32)  [unwired: 1 in]
            n175 = local read "Clave"() -> (w305:string)
            n176 = Equal?(x="admin", y=w299) -> (x = y?=w314:bool)
            n177 = Index Array(array=w307, index=w306) -> (element=w304:string)
            n178 = Equal?(x="Ab123456", y=w305) -> (x = y?=w313:bool)
            n179 = Equal?(x=w305, y=w304) -> (x = y?=w303:bool)
            n180 = And(x=w314, y=w313) -> (x .and. y?=w312:bool)
            n181 = Select(t=Control_1."Inicio", s=w303, f=Control_1."Login") -> (s? t:f=w300:T1)
            n182 = Select(t=Control_1."Registro", s=w312, f=w300) -> (s? t:f=w310:T1)
          }
        }
      }
      frame "Registro" {
        n183 = call-poly <vilib>:"Read Delimited Spreadsheet.vi"("file path (dialog if empty)"=w322, "format (%s)"="%s", "delimiter (\\t)"="\t") -> ("all rows"=w319:string[][])  [unwired: 7 in, 5 out]
        n184 = local write "Tab Control"(enum32{"Login", "Registro", "Inicio"}."Registro" ("Tab Control")) -> ()
        n185 = Index Array(array=w319, index (col) #1=0 ("disabled index (col)"), index (col) #2=1 ("index (col)")) -> (element #1=w318:string[], element #2=w317:string[])  [unwired: 2 in]
        n186 = event shown="[2] \"Volver\": Mouse Up" {
          selector: _ -> [_ _ _]
          dyn-events: _ -> [_ _ _]
          timeout: _ -> [_ _ _]
          tunnel: w327 -> [w362 _ _]
          tunnel: w326 -> [w361 _ _]
          tunnel: [Control_1."Registro" Control_1."Registro" Control_1."Login"] -> w325
          tunnel: w318 -> [w358 w426 _]
          tunnel: w317 -> [_ w423 _]
          event "Agregar": Mouse Up {
            # "Caracteres especiales"
            # "Minu"
            # "Num"
            # "Mayusc"
            n187 = event-data() -> ()  [unwired: 1 in, 8 out]
            n188 = local read "Nuevo Usuario"() -> (w337:string)
            n189 = Search 1D Array(1D array=w358, element=w337) -> (index of element=w357:i32)  [unwired: 1 in]
            n190 = String To Byte Array(string=w337) -> (unsigned byte array=w353:u8[])
            n191 = String To Byte Array(string=w337) -> (unsigned byte array=w348:u8[])
            n192 = String To Byte Array(string=w337) -> (unsigned byte array=w347:u8[])
            n193 = String To Byte Array(string=w337) -> (unsigned byte array=w338:u8[])
            n194 = local read "Clave Nueva"() -> (w359:string)
            n195 = In Range and Coerce(upper limit=u8 48, x=w353, lower limit=u8 32) -> (In Range?=w344:bool[])  [unwired: 1 out]
            n196 = Not Equal?(x=w357, y=-1) -> (x != y?=w355:bool)
            n197 = In Range and Coerce(upper limit=u8 65, x=w348, lower limit=u8 58) -> (In Range?=w343:bool[])  [unwired: 1 out]
            n198 = In Range and Coerce(upper limit=u8 97, x=w347, lower limit=u8 91) -> (In Range?=w342:bool[])  [unwired: 1 out]
            n199 = In Range and Coerce(upper limit=u8 255, x=w338, lower limit=u8 123) -> (In Range?=w341:bool[])  [unwired: 1 out]
            n200 = Equal?(x=w337, y=w359) -> (x = y?=w367:bool)
            n201 = Or Array Elements(Boolean array=w343) -> (logical OR=w335:bool)
            n202 = Or Array Elements(Boolean array=w342) -> (logical OR=w334:bool)
            n203 = Or Array Elements(Boolean array=w341) -> (logical OR=w333:bool)
            n204 = String Length(string=w359) -> (length=w389:i32)
            n205 = String Length(string=w359) -> (length=w387:i32)
            n206 = String To Byte Array(string=w359) -> (unsigned byte array=w375:u8[])
            n207 = String To Byte Array(string=w359) -> (unsigned byte array=w376:u8[])
            n208 = String To Byte Array(string=w359) -> (unsigned byte array=w383:u8[])
            n209 = Or Array Elements(Boolean array=w344) -> (logical OR=w336:bool)
            n210 = Not(x=w333) -> (.not. x?=w329:bool)
            n211 = Greater Or Equal?(x=w387, y=8) -> (x >= y?=w384:bool)
            n212 = Less Or Equal?(x=w389, y=16) -> (x <= y?=w385:bool)
            n213 = In Range and Coerce(upper limit=u8 90, x=w375, lower limit=u8 65) -> (In Range?=w372:bool[])  [unwired: 1 out]
            n214 = In Range and Coerce(upper limit=u8 57, x=w376, lower limit=u8 48) -> (In Range?=w379:bool[])  [unwired: 1 out]
            n215 = In Range and Coerce(upper limit=u8 122, x=w383, lower limit=u8 97) -> (In Range?=w380:bool[])  [unwired: 1 out]
            n216 = Or Array Elements(Boolean array=w372) -> (logical OR=w370:bool)
            n217 = Or Array Elements(Boolean array=w379) -> (logical OR=w369:bool)
            n218 = Or Array Elements(Boolean array=w380) -> (logical OR=w368:bool)
            n219 = And(x=w385, y=w384) -> (x .and. y?=w371:bool)
            n220 = Not(x=w355) -> (.not. x?=w354:bool)
            n221 = Not(x=w367) -> (.not. x?=w366:bool)
            n222 = Not(x=w336) -> (.not. x?=w332:bool)
            n223 = Not(x=w335) -> (.not. x?=w331:bool)
            n224 = Not(x=w334) -> (.not. x?=w330:bool)
            n225 = Compound Arithmetic op=AND(w354, w366, w371, w370, w369, w368, w332, w331, w330, w329) -> (w365:bool)
            n226 = case shown="True" w365 {
              selector: w365 -> [w398 _]
              tunnel: [w393 w407] -> w364
              tunnel: [w392 w406] -> w363
              tunnel: w362 -> [w393 w404]
              tunnel: w361 -> [w392 w403]
              frame False {
                n227 = Not(x=w398) -> (.not. x?=w397:bool)
                n228 = local write "concatenated string"("" ("concatenated string")) -> ()
                n229 = property on="concatenated string" class="Str"("Visible"=w397) -> ()  [unwired: 2 in, 2 out]
                n230 = Concatenate Strings("*El usuario o la contraseña son incorrectas", "\n\n" ("string"), "*La contraseña tiene que ser diferente al usuario; debe tener una\nletra mayuscula, una letra minuscula y un número", "\n\n" ("string"), "*La clave debe ser mayor o igual a 8 (Ocho) caracteres y \nmenor a 16 (Dieciseis) caracteres", "\n\n" ("string"), "*El usuario  está repetido") -> (→"concatenated string":string)
              }
              frame True {
                n231 = local read "Nuevo Usuario"() -> (w410:string)
                n232 = property on="concatenated string" class="Str"("Visible"=FALSE) -> ()  [unwired: 2 in, 2 out]
                n233 = Set File Position(refnum=w404, from (0:start)=enum16{"start", "end", "current"}."end", error in=w403) -> (refnum out=w408:refnum<file>, error out=w413:errorcluster)  [unwired: 1 in]
                n234 = local read "Clave Nueva"() -> (w411:string)
                n235 = Concatenate Strings(w410, "\t", w411, "\r\n") -> (w414:string)
                n236 = Write to Text File(file (use dialog)=w408, text=w414, error in=w413) -> (refnum out=w407:refnum<file>, error out=w406:errorcluster)  [unwired: 1 in, 1 out]
              }
            }
            n237 = Close File(refnum=w364, error in=w363) -> ()  [unwired: 2 out]
          }
          event "Borrar": Mouse Up {
            n238 = event-data() -> ()  [unwired: 1 in, 8 out]
            n239 = local read "Borrar usuario"() -> (w416:string)
            n240 = local write "Tab Control"(enum32{"Login", "Registro", "Inicio"}."Registro" ("Tab Control")) -> ()
            n241 = Equal?(x=w416, y="admin") -> (x = y?=w417:bool)
            n242 = Search 1D Array(1D array=w426, element=w416) -> (index of element=w421:i32)  [unwired: 1 in]
            n243 = Equal?(x=w421, y=-1) -> (x = y?=w419:bool)
            n244 = Or(x=w419, y=w417) -> (x .or. y?=w418:bool)
            n245 = case shown="False" w418 {
              tunnel: w426 -> [_ w448]
              tunnel: w423 -> [_ w447]
              tunnel: w421 -> [_ w446]
              tunnel: w421 -> [_ w445]
              frame True {
                n246 = property on="String" class="Str"("Visible"=TRUE) -> ()  [unwired: 2 in, 2 out]
                "String" <- "**Usuario incorrecto\n\n**No se puede eliminar admin"
              }
              frame False {
                n247 = Delete From Array(array=w447, index=w446) -> (array with subset deleted=→"Contraseñas":string[])  [unwired: 1 in, 1 out]
                n248 = Delete From Array(array=w448, index=w445) -> (deleted portion=w430:string, array with subset deleted=w442:string[])  [unwired: 1 in]
                "Usuarios" <- w442
                n249 = call <vilib>:"Application Directory.vi"() -> ("Application Directory"=w435:path)
                n250 = Build Path(base path=w435, name or relative path=path "usuario.txt" ("file path (use dialog)")) -> (appended path=w436:path)
                n251 = Array Size(array=w442) -> (size(s)=w441:i32)
                n252 = Open/Create/Replace File(file path (use dialog)=w436, operation (0:open)=T2."replace or create", access (0:read/write)=enum16{"read/write", "read-only", "write-only"}."read/write") -> (refnum out=w433:refnum<file>, error out=w432:errorcluster)  [unwired: 3 in, 1 out]
                n253 = for {
                  N: w441 -> [_]
                  tunnel: [w452] -> w439
                  tunnel: [w451] -> w440
                  tunnel: w433 -> [w450]
                  tunnel: w432 -> [w449]
                  i -> [w461]
                  n254 = local read "Contraseñas"() -> (w462:string[])
                  n255 = local read "Usuarios"() -> (w463:string[])
                  n256 = Index Array(array=w463, index=w461) -> (element=w454:string)
                  n257 = Index Array(array=w462, index=w461) -> (element=w453:string)
                  n258 = Concatenate Strings(w454, "\t", w453, "\r\n") -> (w456:string)
                  n259 = Set File Position(refnum=w450, from (0:start)=enum16{"start", "end", "current"}."end", error in=w449) -> (refnum out=w458:refnum<file>, error out=w460:errorcluster)  [unwired: 1 in]
                  n260 = Write to Text File(file (use dialog)=w458, text=w456, error in=w460) -> (refnum out=w451:refnum<file>, error out=w452:errorcluster)  [unwired: 1 in, 1 out]
                }
                n261 = local read "Usuarios Eliminados"() -> (w431:string[])
                n262 = Insert Into Array(array=w431, new element=w430) -> (w429:string[])  [unwired: 1 in]
                n263 = local write "Usuarios Eliminados"(w429) -> ()
                n264 = property on="String" class="Str"("Visible"=FALSE) -> ()  [unwired: 2 in, 2 out]
                n265 = Close File(refnum=w440, error in=w439) -> ()  [unwired: 2 out]
              }
            }
          }
          event "Volver": Mouse Up {
            n266 = event-data() -> ()  [unwired: 1 in, 8 out]
            n267 = local write "Tab Control"(enum32{"Login", "Registro", "Inicio"}."Login" ("Tab Control")) -> ()
          }
        }
      }
      frame "Inicio" {
        n268 = local write "Tab Control"(enum32{"Login", "Registro", "Inicio"}."Inicio" ("Tab Control")) -> ()
        n269 = local read "Usuario"() -> (w468:string)
        n270 = Dequeue Element(queue=w470, error in (no error)=w469) -> (element=w467:string)  [unwired: 1 in, 3 out]
        n271 = Equal?(x=w468, y=w467) -> (x = y?=w466:bool)
        n272 = case shown="True" w466 {
          frame False {
          }
          frame True {
            n273 = property on="OK Button 4" class="Bool (strict)"() -> ("Value"=w473:bool)  [unwired: 2 in, 2 out]
            n274 = Not(x=w473) -> (.not. x?=w474:bool)
            n275 = property on="OK Button 4" class="Bool (strict)"("Val(Sgnl)"=w474) -> ()  [unwired: 2 in, 2 out]
          }
        }
        n276 = event shown="[1] \"OK Button 4\": Value Change" {
          selector: _ -> [_ _]
          dyn-events: _ -> [_ _]
          timeout: _ -> [_ _]
          tunnel: [Control_1."Login" Control_1."Login"] -> w471
          event "Cerrar sesión": Mouse Up {
            n277 = event-data() -> ()  [unwired: 1 in, 8 out]
            n278 = local write "Tab Control"(enum32{"Login", "Registro", "Inicio"}."Login" ("Tab Control")) -> ()
          }
          event "OK Button 4": Value Change {
            n279 = event-data() -> ()  [unwired: 1 in, 6 out]
            n280 = local write "Tab Control 2"(enum32{"Login", "Registro", "Inicio"}."Login" ("Tab Control")) -> ()
          }
        }
      }
    }
    n281 = node-c288() -> ()  [unwired: 1 in, 1 out]
  }
  n282 = node-c288(w23) -> ()  [unwired: 1 out]
  n283 = node-c288(w54) -> ()  [unwired: 1 out]
  "Usuarios Eliminados" <- string[] [] ("Usuarios Eliminados")
